vi "Asylum_CloseRefnum.vi"(8 "error in (no error)":errorcluster, 11 "Application":refnum<k7>) -> (0 "error out":errorcluster)   [LabVIEW 2020]
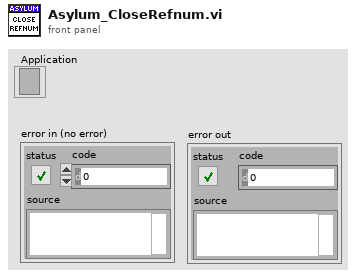
[diagram p1: front panel]
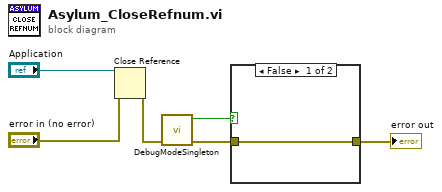
[diagram p0: block diagram]
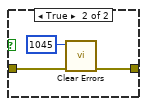
[diagram p2: hidden frame]
diagram:
  n1 = Close Reference(reference="Application", error in (no error)="error in (no error)") -> (error out=w2:errorcluster)
  n2 = call "DebugModeSingleton.vi"() -> ("Debug Mode?"=w3:bool)  [unwired: 11 in]
  n3 = case shown="False" w3 {
    tunnel: w2 -> [w6 w9]
    tunnel: [w6 w8] -> w1
    frame False {
    }
    frame True {
      n4 = call <vilib>:"Clear Errors.vi"("error in (no error)"=w9, "specific error code to clear (0: all)"=1045) -> ("error out"=w8:errorcluster)  [unwired: 4 in, 1 out]
    }
  }
  "error out" <- w1
